vi "LIA Simulator.vi"() -> ()   [LabVIEW 2018]
uses:
  <vilib>/Analysis/4window.llb/windowTd.ctl
  <vilib>/Analysis/5stat.llb/RMS (DBL).vi
  <vilib>/Analysis/2dsp.llb/Decimate (single shot, CDB).vi
  <vilib>/measure/maspectr.llb/FFT Power Spectrum and PSD for 1 Chan (CDB).vi
  <vilib>/measure/maspectr.llb/FFT Power Spectrum and PSD for 1 Chan.vi
  <vilib>/addons/Digital Filter Design/Analysis.llb/DFD Plot Freq Response (Linear-Spaced).vi
  <vilib>/addons/Digital Filter Design/Process.llb/DFD Filtering (Array).vi
  <vilib>/measure/NI_MAPro.lvlib
  <vilib>/Analysis/NI_AALPro.lvlib
  <vilib>/addons/Digital Filter Design/NI_DigFilterLicensed.lvlib
  <vilib>/Analysis/NI_AALBase.lvlib
panel:
  out "Noise power":dbl format="%#_p"
  in  "BW":dbl=100000.0 format="%#_13p"
  in  "5783 AND nV/sqrt(Hz)":dbl=1.8e-08 format="%#_13p"
  in  "Iterations":i32=100
  out "FFT Gain":dbl
  out "Audio Depth":dbl format="%#_p"
  in  "Resolution":dbl=19.0 format="%#_13g"
  in  "Sampling Rate":dbl=1.0 format="%#_p"
  in  "Number Samples":i32=10000
  out "Error Out":errorcluster
  in  "Error In":errorcluster
  in  "Stop":bool
  in  "Tab Control 3":T1(tab)
  out "Noise vrms":dbl
  out "Noise (W|50ohms)":dbl
  out "k":dbl
  out "Pavg 0":dbl format="%0.2p"
  out "std dev 0":dbl format="%0.2p"
  out "mean0":dbl format="%0.2p"
  out "mean1":dbl format="%0.2p"
  out "std dev 1":dbl format="%0.2p"
  out "Pavg 1":dbl format="%0.2p"
  out "mean 2":dbl format="%0.2p"
  out "std dev 2":dbl format="%0.2p"
  out "Pavg 2":dbl format="%0.2p"
  out "IIR Filter Cluster":T2
  out "gain":dbl
  out "structure":u16(ring) items=["Invalid", "FIR Direct Form", "FIR Direct Form Transposed", "FIR Symmetric", "FIR Antisymmetric", "IIR Direct Form I", "IIR Direct Form I Transposed", "IIR Direct Form II", "IIR Direct Form II Transposed", "IIR Cascaded Second-Order Sections Form I", "IIR Cascaded Second-Order Sections Form I Transposed", "IIR Cascaded Second-Order Sections Form II", "IIR Cascaded Second-Order Sections Form II Transposed", "Lattice Allpass (basic sections)", "Lattice Allpass (one multiplier sections)", "Lattice Allpass (normalized sections)", "Lattice AR (basic sections)", "Lattice AR (one multiplier sections)", "Lattice AR (normalized sections)", "Lattice MA (minimum phase)", "Lattice MA (maximum phase)", "Lattice ARMA (basic sections)", "Lattice ARMA (one multiplier sections)", "Lattice ARMA (normalized sections)"]
  out "mean 3":dbl format="%0.2p"
  out "std dev 3":dbl format="%0.2p"
  out "Pavg 3":dbl format="%0.2p"
  in  "Tab Control 2":T3(tab)
  out "Oscillator IQ":dbl[][](graph)
  out "Oscillator Spectrum":cluster{"f0":dbl, "df":dbl, "magnitude":dbl[]}(graph)
  out "Waveform Graph 8":dbl[](graph)
  out "Waveform Graph 7":cluster{"f0":dbl, "df":dbl, "magnitude":dbl[]}(graph)
  out "Waveform Graph 10":dbl[](graph)
  out "Waveform Graph 9":cluster{"f0":dbl, "df":dbl, "magnitude":dbl[]}(graph)
  out "Waveform Graph 12":dbl[](graph)
  out "Waveform Graph 11":cluster{"f0":dbl, "df":dbl, "magnitude":dbl[]}(graph)
  out "Waveform Graph 14":dbl[][](graph)
  out "Waveform Graph 13":cluster{"f0":dbl, "df":dbl, "magnitude":dbl[]}(graph)
  out "Waveform Graph 17":cluster{"f0":dbl, "df":dbl, "values":dbl[]}[](graph)
  out "Waveform Graph 16":dbl[](graph)
  out "Waveform Graph 15":cluster{"f0":dbl, "df":dbl, "magnitude":dbl[]}(graph)
  out "Waveform Graph 20":dbl[](graph)
  out "Waveform Graph 19":cluster{"f0":dbl, "df":dbl, "magnitude":dbl[]}(graph)
  out "Waveform Graph 23":dbl[](graph)
  out "Waveform Graph 22":cluster{"f0":dbl, "df":dbl, "magnitude":dbl[]}(graph)
  in  "Tab Control 1":T4(tab)
  in  "Oscillator Frequency":dbl=0.001 format="%#_p"
  in  "Oscillator Magnitude":dbl=1.0 format="%#_13g"
  in  "Signal Frequency":dbl=0.001 format="%#_p"
  in  "Signal Offset":cdb format="%#_13g"
  in  "Singal Amplitude":dbl=1.0 format="%#_13g"
  in  "Desired SNR (dB)":dbl=70.0 format="%#_p"
  in  "Decimation 1":i32=5
  in  "beta":dbl=10.0 format="%.2f"
  in  "low cutoff freq [Hz] 1":dbl=0.05
  in  "Filter delay 1":i32=50
  in  "Decimation 2":i32=4
  in  "stopband atten [dB] 2":dbl=60.0 format="%.2f"
  in  "low cutoff freq [Hz] 2":dbl=0.0005
  in  "Filter delay 2":i32=100
  in  "low cutoff freq [Hz] 3":dbl=0.0001 format="%#_p"
  in  "beta 3":dbl=12.0 format="%.2f"
  in  "Decimation 3":i32=32
  in  "Filter delay 3":i32=150
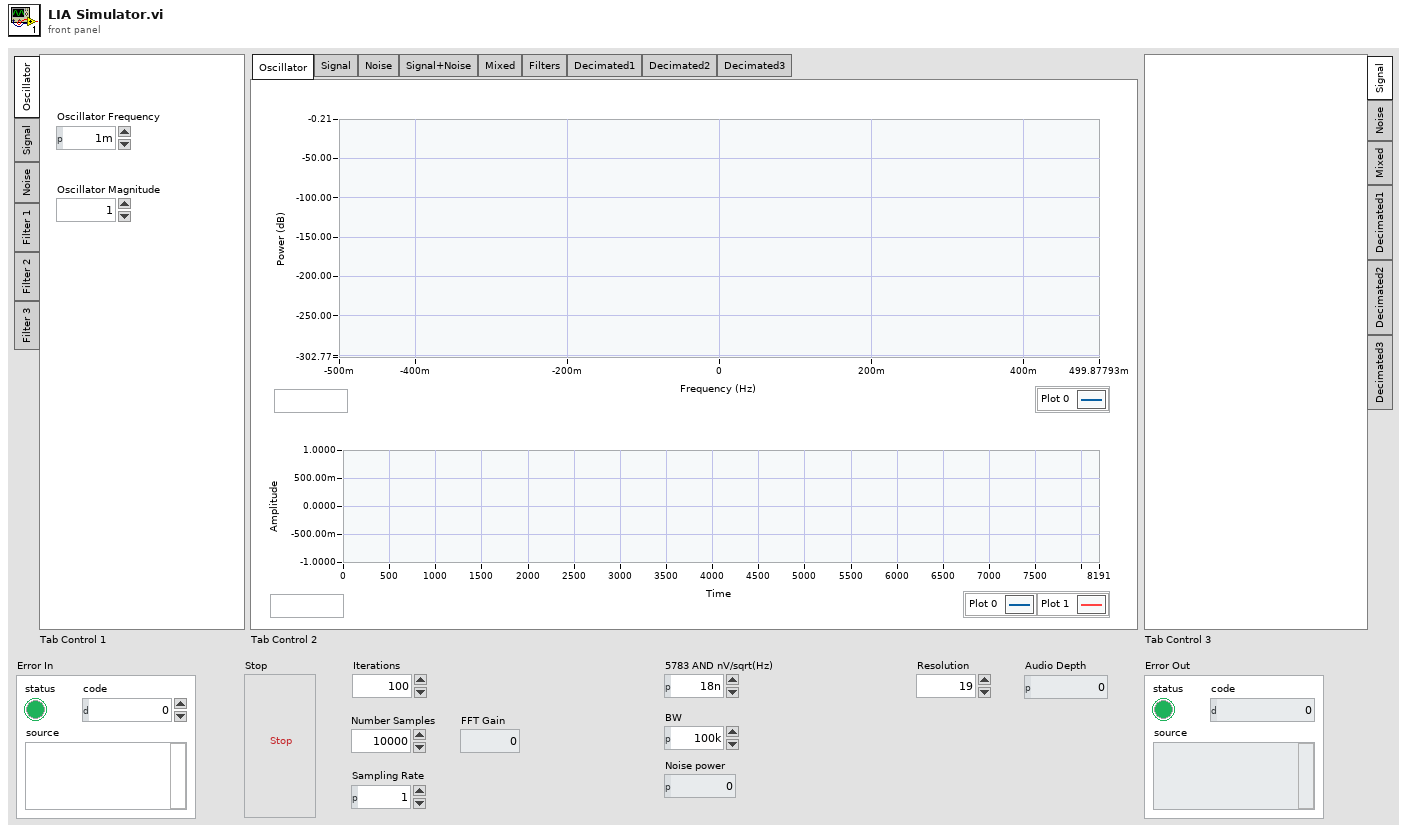
[diagram p1: front panel]
types:
  T1 = enum32{"Signal", "Noise", "Mixed", "Decimated1", "Decimated2", "Decimated3"}
  T2 = cluster{"filter structure":enum32{"IIR 2nd Order", "IIR 4th Order"}, "Reverse Coefficients":dbl[], "Forward Coefficients":dbl[]}
  T3 = enum32{"Oscillator", "Signal", "Noise", "Signal+Noise", "Mixed", "Filters", "Decimated1", "Decimated2", "Decimated3"}
  T4 = enum32{"Oscillator", "Signal", "Noise", "Filter 1", "Filter 2", "Filter 3"}
  T5 = cluster{"averaging mode":enum16{"No averaging", "Vector averaging", "RMS averaging", "Peak hold"}, "weighting mode":enum16{"Linear", "Exponential"}, "number of averages":u32}
  T6 = typedef "NI_AALPro.lvlib/windowTd.ctl" = u32
  T7 = typedef "NI_DigFilterLicensed.lvlib/DFD Filter Obj.ctl" = cluster{"mSRate_Fs":dbl, "mSRate_Version":string, "mSRate_Comments":string, "mSRate_OrgCoef":T8, "mSRate_CurCoef":T8, "mSRate_Quantized?":bool, "mSRate_QCoef":T8, "mSRate_QSettings":T10[], "mSRate_Order":i32, "mSRate_Scaling":cluster{"mSRate_ScaleByPowerOf2?":bool, "mSRate_ScaleType":T12}}
  T8 = typedef "NI_DigFilterLicensed.lvlib/DFD Filter Coef.ctl" = cluster{"type":T9, "gain":dbl, "coef a (k)":dbl[], "coef b (v)":dbl[]}
  T9 = typedef "NI_DigFilterLicensed.lvlib/DFD Filter Structure Type Selector.ctl" = enum16{"Undefined", "FIR Direct Form", "FIR Direct Form Transposed", "FIR Symmetric", "FIR Antisymmetric", "IIR Direct Form I", "IIR Direct Form I Transposed", "IIR Direct Form II", "IIR Direct Form II Transposed", "IIR Cascaded Second Order Sections Form I", "IIR Cascaded Second Order Sections Form I Transposed", "IIR Cascaded Second Order Sections Form II", "IIR Cascaded Second Order Sections Form II Transposed", "Lattice Allpass (basic sections)", "Lattice Allpass (one multiplier sections)", "Lattice Allpass (normalized sections)", "Lattice AR (basic sections)", "Lattice AR (one multiplier sections)", "Lattice AR (normalized sections)", "Lattice MA (minimum phase)", "Lattice MA (maximum phase)", "Lattice ARMA (basic sections)", "Lattice ARMA (one multiplier sections)", "Lattice ARMA (normalized sections)"}
  T10 = typedef "NI_DigFilterLicensed.lvlib/dfd_Internal Quantization Settings.ctl" = cluster{"source":T11, "wl":i16, "iwl":i16, "overflow mode":enum16{"Saturation", "Wrap"}, "rounding mode":enum16{"Nearest", "Truncation"}, "signed?":bool}
  T11 = typedef "NI_DigFilterLicensed.lvlib/dfd_Internal Quantization Srcs.ctl" = u16
  T12 = typedef "NI_DigFilterLicensed.lvlib/DFD Coef Norm Type.ctl" = enum16{"No Norm", "Time Domain 1-Norm", "Time Domain 2-Norm", "Time Domain Inf-Norm"}
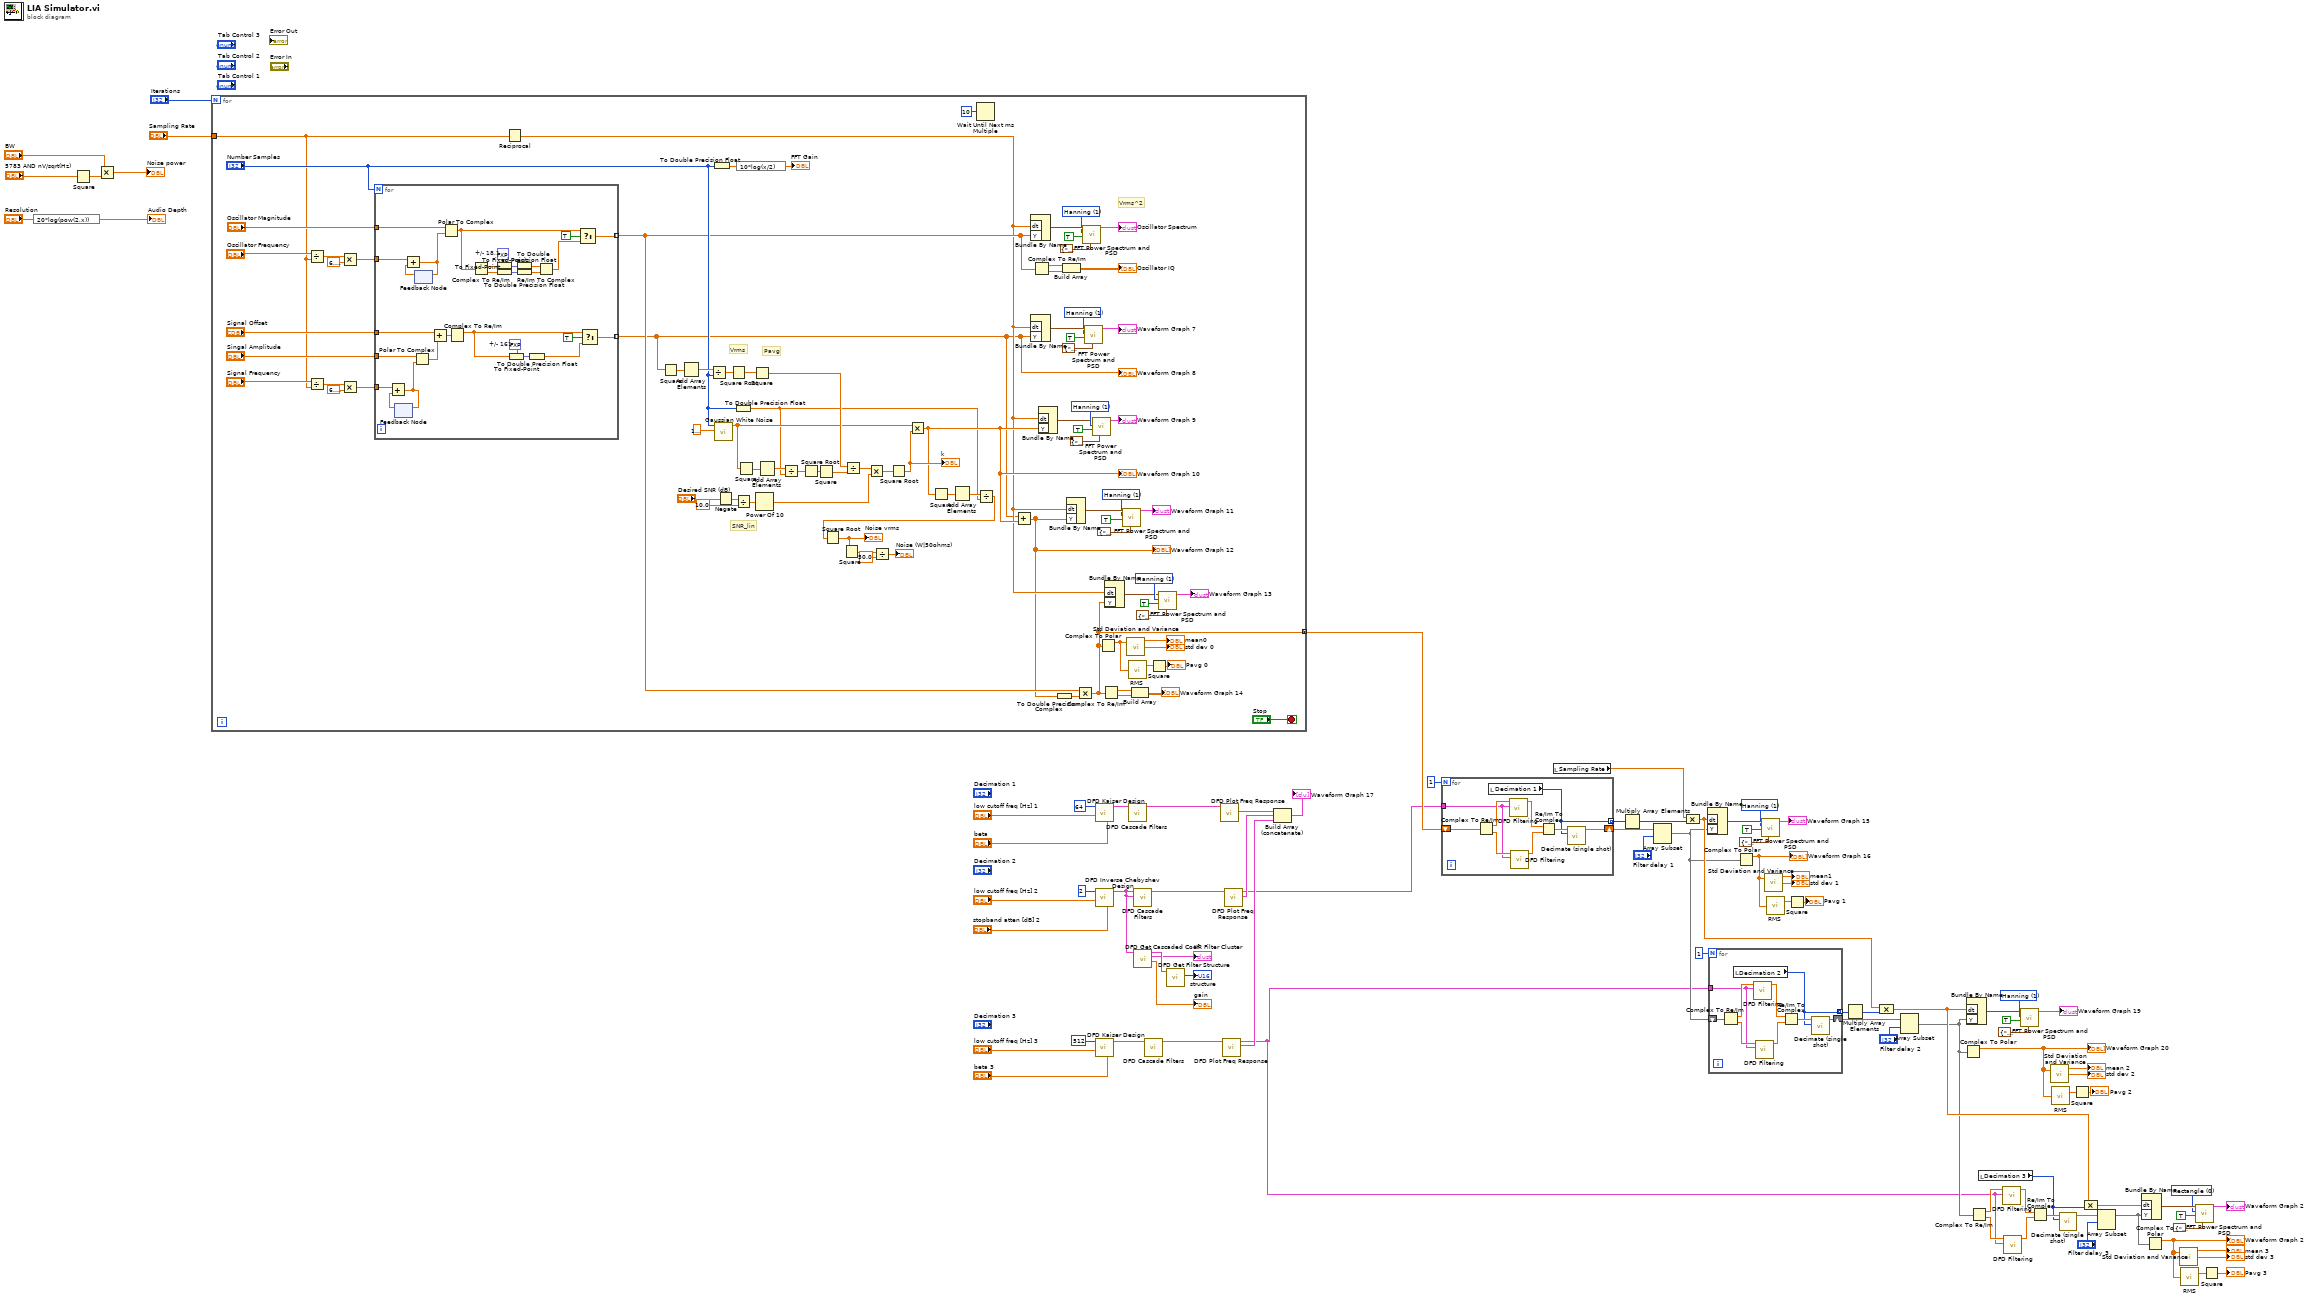
[diagram p0: block diagram]
diagram:
  w34 = T6 0 items=["Rectangle"=0, "Hanning"=1, "Hamming"=2, "Blackman-Harris"=3, "Exact Blackman"=4, "Blackman"=5, "Flat Top"=6, "4 Term B-Harris "=7, "7 Term B-Harris"=8, "Low Sidelobe"=9, "Blackman Nuttall"=11, "Triangle"=30, "Bartlett-Hanning"=31, "Bohman"=32, "Parzen"=33, "Welch"=34, "Kaiser"=60, "Dolph-Chebyshev"=61, "Gaussian"=62] ("window")
  w70 = T6 1 items=["Rectangle"=0, "Hanning"=1, "Hamming"=2, "Blackman-Harris"=3, "Exact Blackman"=4, "Blackman"=5, "Flat Top"=6, "4 Term B-Harris "=7, "7 Term B-Harris"=8, "Low Sidelobe"=9, "Blackman Nuttall"=11, "Triangle"=30, "Bartlett-Hanning"=31, "Bohman"=32, "Parzen"=33, "Welch"=34, "Kaiser"=60, "Dolph-Chebyshev"=61, "Gaussian"=62] ("window")
  w71 = T6 1 items=["Rectangle"=0, "Hanning"=1, "Hamming"=2, "Blackman-Harris"=3, "Exact Blackman"=4, "Blackman"=5, "Flat Top"=6, "4 Term B-Harris "=7, "7 Term B-Harris"=8, "Low Sidelobe"=9, "Blackman Nuttall"=11, "Triangle"=30, "Bartlett-Hanning"=31, "Bohman"=32, "Parzen"=33, "Welch"=34, "Kaiser"=60, "Dolph-Chebyshev"=61, "Gaussian"=62] ("window")
  n1 = expression code="20*log(pow(2,x))"("Resolution") -> (→"Audio Depth":dbl)
  n2 = Square(x="5783 AND nV/sqrt(Hz)") -> (x^2=w82:dbl)
  n3 = Multiply(x="BW", y=w82) -> (x*y=→"Noise power":dbl)
  n4 = for {
    N: "Iterations" -> [_]
    tunnel: "Sampling Rate" -> [w101]
    tunnel: [w94] -> w59 mode=concatenating
    stop <- "Stop" stop-if-true
    w110 = T6 1 items=["Rectangle"=0, "Hanning"=1, "Hamming"=2, "Blackman-Harris"=3, "Exact Blackman"=4, "Blackman"=5, "Flat Top"=6, "4 Term B-Harris "=7, "7 Term B-Harris"=8, "Low Sidelobe"=9, "Blackman Nuttall"=11, "Triangle"=30, "Bartlett-Hanning"=31, "Bohman"=32, "Parzen"=33, "Welch"=34, "Kaiser"=60, "Dolph-Chebyshev"=61, "Gaussian"=62] ("window")
    w118 = T6 1 items=["Rectangle"=0, "Hanning"=1, "Hamming"=2, "Blackman-Harris"=3, "Exact Blackman"=4, "Blackman"=5, "Flat Top"=6, "4 Term B-Harris "=7, "7 Term B-Harris"=8, "Low Sidelobe"=9, "Blackman Nuttall"=11, "Triangle"=30, "Bartlett-Hanning"=31, "Bohman"=32, "Parzen"=33, "Welch"=34, "Kaiser"=60, "Dolph-Chebyshev"=61, "Gaussian"=62] ("window")
    w158 = T6 1 items=["Rectangle"=0, "Hanning"=1, "Hamming"=2, "Blackman-Harris"=3, "Exact Blackman"=4, "Blackman"=5, "Flat Top"=6, "4 Term B-Harris "=7, "7 Term B-Harris"=8, "Low Sidelobe"=9, "Blackman Nuttall"=11, "Triangle"=30, "Bartlett-Hanning"=31, "Bohman"=32, "Parzen"=33, "Welch"=34, "Kaiser"=60, "Dolph-Chebyshev"=61, "Gaussian"=62] ("window")
    w159 = T6 1 items=["Rectangle"=0, "Hanning"=1, "Hamming"=2, "Blackman-Harris"=3, "Exact Blackman"=4, "Blackman"=5, "Flat Top"=6, "4 Term B-Harris "=7, "7 Term B-Harris"=8, "Low Sidelobe"=9, "Blackman Nuttall"=11, "Triangle"=30, "Bartlett-Hanning"=31, "Bohman"=32, "Parzen"=33, "Welch"=34, "Kaiser"=60, "Dolph-Chebyshev"=61, "Gaussian"=62] ("window")
    w167 = T6 1 items=["Rectangle"=0, "Hanning"=1, "Hamming"=2, "Blackman-Harris"=3, "Exact Blackman"=4, "Blackman"=5, "Flat Top"=6, "4 Term B-Harris "=7, "7 Term B-Harris"=8, "Low Sidelobe"=9, "Blackman Nuttall"=11, "Triangle"=30, "Bartlett-Hanning"=31, "Bohman"=32, "Parzen"=33, "Welch"=34, "Kaiser"=60, "Dolph-Chebyshev"=61, "Gaussian"=62] ("window")
    # "SNR_lin"
    # "Pavg"
    # "Vrms"
    # "Vrms^2"
    n5 = Divide(x="Oscillator Frequency", y=w101) -> (x/y=w154:dbl)
    n6 = Divide(x="Signal Frequency", y=w101) -> (x/y=w175:dbl)
    n7 = Multiply(x=w154, y=6.283185307179586) -> (x*y=w151:dbl)
    n8 = Multiply(x=w175, y=6.283185307179586) -> (x*y=w174:dbl)
    n9 = for {
      N: "Number Samples" -> [_]
      tunnel: w174 -> [w201]
      tunnel: "Singal Amplitude" -> [w204]
      tunnel: "Signal Offset" -> [w203]
      tunnel: [w187] -> w111 mode=indexing
      tunnel: [w181] -> w90 mode=indexing
      tunnel: w151 -> [w192]
      tunnel: "Oscillator Magnitude" -> [w190]
      w182 = fxp<+/-,16,1> 0.0  # +/- 161
      w197 = fxp<+/-,18,1> 0.0  # +/- 18,1
      n10 = feedback #1() -> (w205:dbl)  [unwired: 1 in]
      n11 = Add(x=w201, y=w205) -> (x+y=w200:dbl)
      n12 = feedback-in #1(w200) -> ()
      n13 = Polar To Complex(1:w200, 2:w204) -> (0:w202:cdb)
      n14 = feedback #2() -> (w191:dbl)  [unwired: 1 in]
      n15 = Add(x=w192, y=w191) -> (x+y=w189:dbl)
      n16 = feedback-in #2(w189) -> ()
      n17 = Add(x=w203, y=w202) -> (x+y=w179:cdb)
      n18 = Polar To Complex(1:w189, 2:w190) -> (0:w188:cdb)
      n19 = Complex To Re/Im(x + iy=w179) -> (x=w178:dbl)  [unwired: 1 out]
      n20 = Complex To Re/Im(x + iy=w188) -> (x=w199:dbl, y=w198:dbl)
      n21 = To Fixed-Point(fixed-point type=w197, number=w199) -> (fixed-point=w196:fxp<+/-,18,1>)
      n22 = To Fixed-Point(fixed-point type=w197, number=w198) -> (fixed-point=w195:fxp<+/-,18,1>)
      n23 = To Fixed-Point(fixed-point type=w182, number=w178) -> (fixed-point=w183:fxp<+/-,16,1>)
      n24 = To Double Precision Float(number=w196) -> (double precision float=w194:dbl)
      n25 = To Double Precision Float(number=w195) -> (double precision float=w193:dbl)
      n26 = To Double Precision Float(number=w183) -> (double precision float=w180:dbl)
      n27 = Re/Im To Complex(1:w193, 2:w194) -> (0:w186:cdb)
      n28 = Select(t=w188, s=TRUE, f=w186) -> (s? t:f=w187:cdb)
      n29 = Select(t=w178, s=TRUE, f=w180) -> (s? t:f=w181:dbl)
    }
    "Waveform Graph 8" <- w90
    n30 = Reciprocal(x=w101) -> (1/x=w99:dbl)
    n31 = Square(x=w90) -> (x^2=w149:dbl[])
    n32 = Add Array Elements(numeric array=w149) -> (sum=w148:dbl)
    n33 = Divide(x=w148, y="Number Samples") -> (x/y=w147:dbl)
    n34 = To Double Precision Float(number="Number Samples") -> (double precision float=w114:dbl)
    n35 = call <vilib>:"Gaussian White Noise.vi"("standard deviation"=1.0000000000000002, "samples"="Number Samples") -> ("Gaussian noise pattern"=w131:dbl[])  [unwired: 8 in, 1 out]
    n36 = Negate(x="Desired SNR (dB)") -> (-x=w134:dbl)
    n37 = Square Root(x=w147) -> (sqrt(x)=w146:dbl)
    n38 = To Double Precision Float(number="Number Samples") -> (double precision float=w103:dbl)
    n39 = Divide(x=w134, y=10.0) -> (x/y=w142:dbl)
    n40 = expression code="10*log(x/2)"(w114) -> (→"FFT Gain":dbl)
    n41 = Square(x=w131) -> (x^2=w138:dbl[])
    n42 = Square(x=w146) -> (x^2=w137:dbl)
    n43 = Power Of 10(x=w142) -> (10^x=w133:dbl)
    n44 = Add Array Elements(numeric array=w138) -> (sum=w139:dbl)
    n45 = Divide(x=w139, y=w103) -> (x/y=w140:dbl)
    n46 = Square Root(x=w140) -> (sqrt(x)=w141:dbl)
    n47 = Square(x=w141) -> (x^2=w136:dbl)
    n48 = Divide(x=w137, y=w136) -> (x/y=w135:dbl)
    n49 = Multiply(x=w135, y=w133) -> (x*y=w132:dbl)
    n50 = Square Root(x=w132) -> (sqrt(x)=w130:dbl)
    "k" <- w130
    n51 = Multiply(x=w131, y=w130) -> (x*y=w117:dbl[])
    "Waveform Graph 10" <- w117
    n52 = Square(x=w117) -> (x^2=w129:dbl[])
    n53 = Add Array Elements(numeric array=w129) -> (sum=w128:dbl)
    n54 = Wait Until Next ms Multiple(millisecond multiple=u32 10) -> ()  [unwired: 1 out]
    n55 = Divide(x=w128, y=w103) -> (x/y=w127:dbl)
    n56 = Square Root(x=w127) -> (sqrt(x)=w126:dbl)
    "Noise vrms" <- w126
    n57 = Square(x=w126) -> (x^2=w125:dbl)
    n58 = Divide(x=w125, y=50.0) -> (x/y=→"Noise (W|50ohms)":dbl)
    n59 = Add(x=w90, y=w117) -> (x+y=w98:dbl[])
    "Waveform Graph 12" <- w98
    n60 = Bundle By Name("dt"=w99, "Y"=w111) -> (w170:waveform(cdb))  [unwired: 1 in]
    n61 = Bundle By Name("dt"=w99, "Y"=w90) -> (w162:waveform(dbl))  [unwired: 1 in]
    n62 = Complex To Re/Im(x + iy=w111) -> (x=w165:dbl[], y=w164:dbl[])
    n63 = Bundle By Name("dt"=w99, "Y"=w117) -> (w155:waveform(dbl))  [unwired: 1 in]
    n64 = To Double Precision Complex(1:w98) -> (0:w97:cdb[])
    n65 = Build Array(w165, w164) -> (→"Oscillator IQ":dbl[][])
    n66 = Bundle By Name("dt"=w99, "Y"=w98) -> (w121:waveform(dbl))  [unwired: 1 in]
    n67 = Multiply(x=w111, y=w97) -> (x*y=w94:cdb[])
    n68 = call-poly <vilib>:"FFT Power Spectrum and PSD.vi"("averaging parameters"=T5 {"averaging mode"=enum."No averaging", "weighting mode"=enum."Exponential", "number of averages"=10}, "dB On (F)"=TRUE, "window"=w167, "time signal"=w170) -> ("Power Spectrum / PSD"=→"Oscillator Spectrum":cluster{"f0":dbl, "df":dbl, "magnitude":dbl[]})  [unwired: 4 in, 3 out]
    n69 = call-poly <vilib>:"FFT Power Spectrum and PSD.vi"("averaging parameters"=T5 {"averaging mode"=enum."RMS averaging", "weighting mode"=enum."Exponential", "number of averages"=10}, "dB On (F)"=TRUE, "window"=w159, "time signal"=w162) -> ("Power Spectrum / PSD"=→"Waveform Graph 7":cluster{"f0":dbl, "df":dbl, "magnitude":dbl[]})  [unwired: 4 in, 3 out]
    n70 = call-poly <vilib>:"FFT Power Spectrum and PSD.vi"("averaging parameters"=T5 {"averaging mode"=enum."RMS averaging", "weighting mode"=enum."Exponential", "number of averages"=10}, "dB On (F)"=TRUE, "window"=w158, "time signal"=w155) -> ("Power Spectrum / PSD"=→"Waveform Graph 9":cluster{"f0":dbl, "df":dbl, "magnitude":dbl[]})  [unwired: 4 in, 3 out]
    n71 = Complex To Polar(r * e^(i*theta)=w94) -> (r=w93:dbl[])  [unwired: 1 out]
    n72 = Complex To Re/Im(x + iy=w94) -> (x=w105:dbl[], y=w106:dbl[])
    n73 = Bundle By Name("dt"=w99, "Y"=w94) -> (w107:waveform(cdb))  [unwired: 1 in]
    n74 = call-poly <vilib>:"FFT Power Spectrum and PSD.vi"("averaging parameters"=T5 {"averaging mode"=enum."RMS averaging", "weighting mode"=enum."Exponential", "number of averages"=10}, "dB On (F)"=TRUE, "window"=w118, "time signal"=w121) -> ("Power Spectrum / PSD"=→"Waveform Graph 11":cluster{"f0":dbl, "df":dbl, "magnitude":dbl[]})  [unwired: 4 in, 3 out]
    n75 = call <vilib>:"Std Deviation and Variance.vi"("X"=w93) -> ("mean"=→"mean0":dbl, "standard deviation"=→"std dev 0":dbl)  [unwired: 1 in, 1 out]
    n76 = call-poly <vilib>:"RMS.vi"("X"=w93) -> ("rms value"=w92:dbl)  [unwired: 1 out]
    n77 = Build Array(w105, w106) -> (→"Waveform Graph 14":dbl[][])
    n78 = Square(x=w92) -> (x^2=→"Pavg 0":dbl)
    n79 = call-poly <vilib>:"FFT Power Spectrum and PSD.vi"("averaging parameters"=T5 {"averaging mode"=enum."RMS averaging", "weighting mode"=enum."Exponential", "number of averages"=10}, "dB On (F)"=TRUE, "window"=w110, "time signal"=w107) -> ("Power Spectrum / PSD"=→"Waveform Graph 13":cluster{"f0":dbl, "df":dbl, "magnitude":dbl[]})  [unwired: 4 in, 3 out]
  }
  n80 = call <vilib>:"DFD Kaiser Design.vi"("beta"="beta", "low cutoff freq [Hz]"="low cutoff freq [Hz] 1", "order"=64) -> ("filter out"=w49:T7)  [unwired: 7 in, 1 out]
  n81 = call <vilib>:"DFD Inverse Chebyshev Design.vi"("stopband atten [dB]"="stopband atten [dB] 2", "low cutoff freq [Hz]"="low cutoff freq [Hz] 2", "order"=2) -> ("filter out"=w6:T7)  [unwired: 7 in, 1 out]
  n82 = call <vilib>:"DFD Kaiser Design.vi"("beta"="beta 3", "low cutoff freq [Hz]"="low cutoff freq [Hz] 3", "order"=512) -> ("filter out"=w45:T7)  [unwired: 7 in, 1 out]
  n83 = call <vilib>:"DFD Cascade Filters.vi"("filter in 1"=w49) -> ("filter out"=w54:T7)  [unwired: 9 in, 1 out]
  n84 = call <vilib>:"DFD Cascade Filters.vi"("filter in 2"=w6, "filter in 1"=w6) -> ("filter out"=w14:T7)  [unwired: 8 in, 1 out]
  n85 = call <vilib>:"DFD Get Cascaded Coef.vi"("filter in"=w6) -> ("gain"=→"gain":dbl, "IIR Filter Cluster"=→"IIR Filter Cluster":T2, "filter out"=w8:T7)  [unwired: 7 in, 1 out]
  n86 = call <vilib>:"DFD Cascade Filters.vi"("filter in 1"=w45) -> ("filter out"=w40:T7)  [unwired: 9 in, 1 out]
  n87 = call <vilib>:"DFD Get Filter Structure.vi"("filter in"=w8) -> ("structure"=→"structure":u16)  [unwired: 8 in, 2 out]
  n88 = call-poly <vilib>:"DFD Plot Freq Response.vi"("filter in"=w54) -> ("magnitude response"=w55:cluster{"f0":dbl, "df":dbl, "values":dbl[]}[])  [unwired: 7 in, 3 out]
  n89 = call-poly <vilib>:"DFD Plot Freq Response.vi"("filter in"=w40) -> ("magnitude response"=w3:cluster{"f0":dbl, "df":dbl, "values":dbl[]}[], "filter out"=w1:T7)  [unwired: 7 in, 2 out]
  n90 = call-poly <vilib>:"DFD Plot Freq Response.vi"("filter in"=w14) -> ("magnitude response"=w4:cluster{"f0":dbl, "df":dbl, "values":dbl[]}[], "filter out"=w2:T7)  [unwired: 7 in, 2 out]
  n91 = Build Array (concatenate)(w55, w4, w3) -> (→"Waveform Graph 17":cluster{"f0":dbl, "df":dbl, "values":dbl[]}[])
  n92 = for {
    N: 1 -> [_]
    tunnel: w2 -> [w207]
    shift-right: [w209] -> w10
    shift-left: w59 -> [w208]
    tunnel: [w206] -> w51 mode=indexing
    n93 = Complex To Re/Im(x + iy=w208) -> (x=w214:dbl[], y=w213:dbl[])
    n94 = local read "Decimation 1"() -> (w206:i32)
    n95 = call-poly <vilib>:"DFD Filtering.vi"("filter"=w207, "signal in"=w214) -> ("signal out"=w212:dbl[])  [unwired: 8 in, 1 out]
    n96 = call-poly <vilib>:"DFD Filtering.vi"("filter"=w207, "signal in"=w213) -> ("signal out"=w211:dbl[])  [unwired: 8 in, 1 out]
    n97 = Re/Im To Complex(1:w211, 2:w212) -> (0:w210:cdb[])
    n98 = call-poly <vilib>:"Decimate (single shot).vi"("decimating factor"=w206, "X"=w210) -> ("Decimated Array"=w209:cdb[])  [unwired: 8 in, 1 out]
  }
  n99 = local read "Sampling Rate"() -> (w74:dbl)
  n100 = Multiply Array Elements(1:w51) -> (0:w48:i32)
  n101 = Array Subset(array=w10, index="Filter delay 1") -> (w9:cdb[])  [unwired: 1 in]
  n102 = Compound Arithmetic op=MULTIPLY(w74, w48) -> (w39:dbl)
  n103 = Bundle By Name("dt"=w39, "Y"=w9) -> (w75:waveform(cdb))  [unwired: 1 in]
  n104 = for {
    N: 1 -> [_]
    tunnel: [w216] -> w60 mode=indexing
    tunnel: w1 -> [w215]
    shift-right: [w217] -> w18
    shift-left: w9 -> [w219]
    n105 = Complex To Re/Im(x + iy=w219) -> (x=w220:dbl[], y=w221:dbl[])
    n106 = local read "Decimation 2"() -> (w216:i32)
    n107 = call-poly <vilib>:"DFD Filtering.vi"("filter"=w215, "signal in"=w220) -> ("signal out"=w222:dbl[])  [unwired: 8 in, 1 out]
    n108 = call-poly <vilib>:"DFD Filtering.vi"("filter"=w215, "signal in"=w221) -> ("signal out"=w223:dbl[])  [unwired: 8 in, 1 out]
    n109 = Re/Im To Complex(1:w223, 2:w222) -> (0:w218:cdb[])
    n110 = call-poly <vilib>:"Decimate (single shot).vi"("decimating factor"=w216, "X"=w218) -> ("Decimated Array"=w217:cdb[])  [unwired: 8 in, 1 out]
  }
  n111 = Complex To Polar(r * e^(i*theta)=w9) -> (r=w56:dbl[])  [unwired: 1 out]
  "Waveform Graph 16" <- w56
  n112 = call-poly <vilib>:"FFT Power Spectrum and PSD.vi"("averaging parameters"=T5 {"averaging mode"=enum."RMS averaging", "weighting mode"=enum."Exponential", "number of averages"=10}, "dB On (F)"=TRUE, "window"=w71, "time signal"=w75) -> ("Power Spectrum / PSD"=→"Waveform Graph 15":cluster{"f0":dbl, "df":dbl, "magnitude":dbl[]})  [unwired: 4 in, 3 out]
  n113 = call <vilib>:"Std Deviation and Variance.vi"("X"=w56) -> ("mean"=→"mean1":dbl, "standard deviation"=→"std dev 1":dbl)  [unwired: 1 in, 1 out]
  n114 = call-poly <vilib>:"RMS.vi"("X"=w56) -> ("rms value"=w57:dbl)  [unwired: 1 out]
  n115 = Square(x=w57) -> (x^2=→"Pavg 1":dbl)
  n116 = Multiply Array Elements(1:w60) -> (0:w41:i32)
  n117 = Compound Arithmetic op=MULTIPLY(w39, w41) -> (w38:dbl)
  n118 = Array Subset(array=w18, index="Filter delay 2") -> (w17:cdb[])  [unwired: 1 in]
  n119 = Complex To Polar(r * e^(i*theta)=w17) -> (r=w19:dbl[])  [unwired: 1 out]
  "Waveform Graph 20" <- w19
  n120 = Bundle By Name("dt"=w38, "Y"=w17) -> (w67:waveform(cdb))  [unwired: 1 in]
  n121 = Complex To Re/Im(x + iy=w17) -> (x=w31:dbl[], y=w30:dbl[])
  n122 = local read "Decimation 3"() -> (w27:i32)
  n123 = call-poly <vilib>:"DFD Filtering.vi"("filter"=w1, "signal in"=w31) -> ("signal out"=w29:dbl[])  [unwired: 8 in, 1 out]
  n124 = call-poly <vilib>:"DFD Filtering.vi"("filter"=w1, "signal in"=w30) -> ("signal out"=w28:dbl[])  [unwired: 8 in, 1 out]
  n125 = call-poly <vilib>:"FFT Power Spectrum and PSD.vi"("averaging parameters"=T5 {"averaging mode"=enum."RMS averaging", "weighting mode"=enum."Exponential", "number of averages"=10}, "dB On (F)"=TRUE, "window"=w70, "time signal"=w67) -> ("Power Spectrum / PSD"=→"Waveform Graph 19":cluster{"f0":dbl, "df":dbl, "magnitude":dbl[]})  [unwired: 4 in, 3 out]
  n126 = Re/Im To Complex(1:w28, 2:w29) -> (0:w32:cdb[])
  n127 = call <vilib>:"Std Deviation and Variance.vi"("X"=w19) -> ("mean"=→"mean 2":dbl, "standard deviation"=→"std dev 2":dbl)  [unwired: 1 in, 1 out]
  n128 = call-poly <vilib>:"RMS.vi"("X"=w19) -> ("rms value"=w53:dbl)  [unwired: 1 out]
  n129 = call-poly <vilib>:"Decimate (single shot).vi"("decimating factor"=w27, "X"=w32) -> ("Decimated Array"=w25:cdb[])  [unwired: 8 in, 1 out]
  n130 = Square(x=w53) -> (x^2=→"Pavg 2":dbl)
  n131 = Compound Arithmetic op=MULTIPLY(w38, w27) -> (w33:dbl)
  n132 = Array Subset(array=w25, index="Filter delay 3") -> (w16:cdb[])  [unwired: 1 in]
  n133 = Bundle By Name("dt"=w33, "Y"=w16) -> (w37:waveform(cdb))  [unwired: 1 in]
  n134 = Complex To Polar(r * e^(i*theta)=w16) -> (r=w23:dbl[])  [unwired: 1 out]
  "Waveform Graph 23" <- w23
  n135 = call <vilib>:"Std Deviation and Variance.vi"("X"=w23) -> ("mean"=→"mean 3":dbl, "standard deviation"=→"std dev 3":dbl)  [unwired: 1 in, 1 out]
  n136 = call-poly <vilib>:"RMS.vi"("X"=w23) -> ("rms value"=w24:dbl)  [unwired: 1 out]
  n137 = call-poly <vilib>:"FFT Power Spectrum and PSD.vi"("averaging parameters"=T5 {"averaging mode"=enum."RMS averaging", "weighting mode"=enum."Exponential", "number of averages"=10}, "dB On (F)"=TRUE, "window"=w34, "time signal"=w37) -> ("Power Spectrum / PSD"=→"Waveform Graph 22":cluster{"f0":dbl, "df":dbl, "magnitude":dbl[]})  [unwired: 4 in, 3 out]
  n138 = Square(x=w24) -> (x^2=→"Pavg 3":dbl)
